vi "Get Ref.vi"(8 "error in (no error)":errorcluster, 11 "Session Handle in":T1) -> (0 "error out":errorcluster, 2 "Ref":refnum<k7>, 3 "Session Handle out":T1)   [LabVIEW 2019, in "HTS.lvlib" / "SequenceFile.lvclass"]
uses:
  SequenceFile.lvclass
  Typedefs/Session Handle.ctl
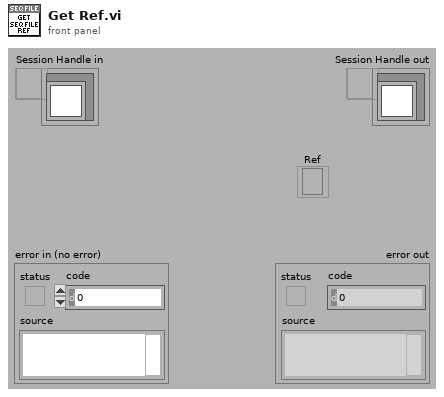
[diagram p1: front panel]
types:
  T1 = typedef "HTS.lvlib/SequenceFile.lvclass/Session Handle.ctl" = refnum<data-value>
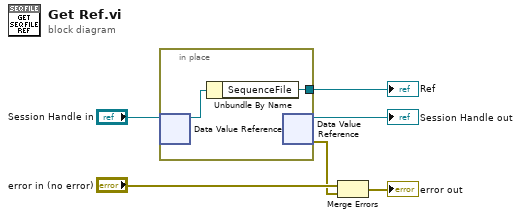
[diagram p0: block diagram]
diagram:
  n1 = in-place {
    in-place-border: [w7] -> w1
    n2 = in-place-dvr #1("Session Handle in") -> (w8:refnum<class "SequenceFile.lvclass">)  [unwired: 1 out]
    n3 = Unbundle By Name(w8) -> ("SequenceFile"=w7:refnum<k7>)
    n4 = in-place-dvr #1() -> (→"Session Handle out":T1, w2:errorcluster)  [unwired: 1 in]
  }
  "Ref" <- w1
  n5 = Merge Errors("error in (no error)", w2) -> (→"error out":errorcluster)
